vi "OpenCVCam_Close.vi"(8 "ErrorIn":errorcluster, 10 "CmdData":variant, 11 "OpenCVCamIn":refnum<class>) -> (0 "ErrorOut":errorcluster, 2 "ReplyData":variant, 3 "OpenCVCamOut":refnum<class>, 4 "Exit":bool)   [LabVIEW 2021, in "OpenCVCam.lvclass"]
uses:
  OpenCVCam.lvclass
  OpenCVCam.lvclass/OpenCVCam.ctl
  State.ctl
  C:/Localdata/Projects/TriekselSoft/TriekselsoftApplicationFramework/Source/.Externals/Library_EmguCV/Emgu.CV.Platform.NetStandard.dll
  Library_EmguCV/Emgu.CV.Platform.NetStandard.dll
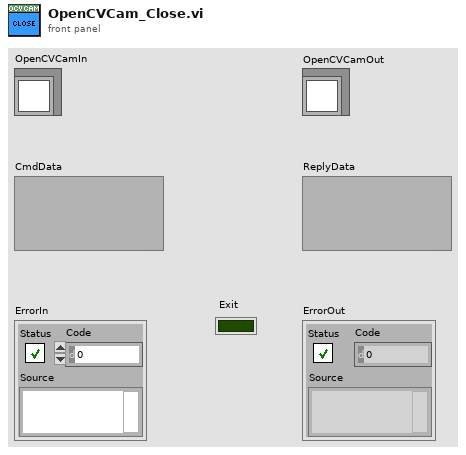
[diagram p1: front panel]
types:
  T1 = typedef "OpenCVCam.lvclass/State.ctl" = enum16{"Idle", "Initialized", "Acquiring"}
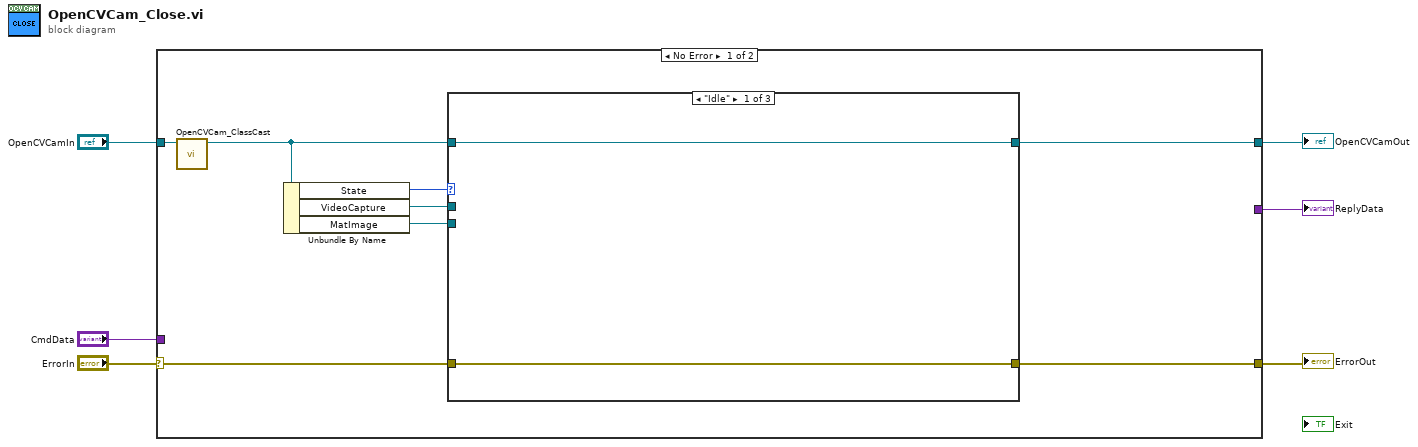
[diagram p0: block diagram]
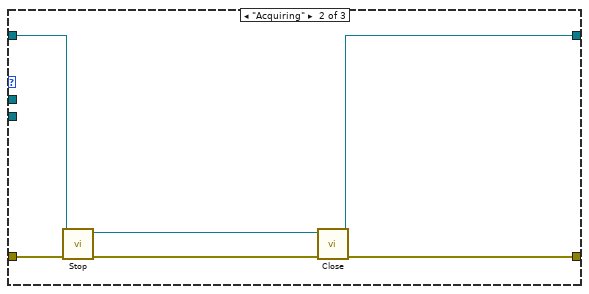
[diagram p2: hidden frame]
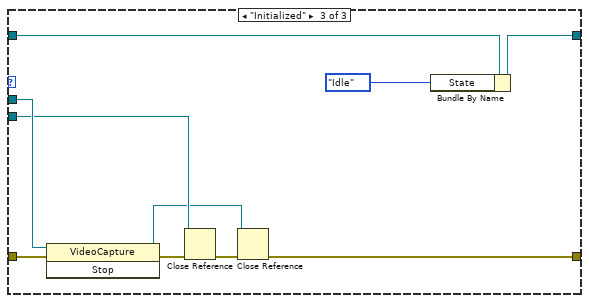
[diagram p3: hidden frame]
diagram:
  n1 = case shown="No Error" "ErrorIn" {
    selector: "ErrorIn" -> [w14 w35]
    tunnel: [w13 w35] -> w5
    tunnel: [_ w34] -> w3
    tunnel: "CmdData" -> [_ w34]
    tunnel: "OpenCVCamIn" -> [w12 w33]
    tunnel: [w7 w33] -> w1
    frame No Error {
      n2 = call "OpenCVCam_ClassCast.vi"("OpenCVCamIn"=w12) -> ("OpenCVCamOut"=w8:refnum<class "OpenCVCam.lvclass">)  [unwired: 10 in]
      n3 = Unbundle By Name(w8) -> ("State"=w11:T1, "VideoCapture"=w10:refnum<k24>, "MatImage"=w9:refnum<k24>)
      n4 = case shown="\"Idle\"" w11 {
        tunnel: [w16 w20 w31] -> w13
        tunnel: w14 -> [w16 w22 w29]
        tunnel: w10 -> [_ _ w28]
        tunnel: w9 -> [_ _ w27]
        tunnel: w8 -> [w15 w19 w25]
        tunnel: [w15 w17 w24] -> w7
        frame "Idle" {
        }
        frame "Acquiring" {
          n5 = call-dynamic "Stop.vi"("ErrorIn"=w22, "OpenCVCamIn"=w19) -> ("ErrorOut"=w21:errorcluster, "OpenCVCamOut"=w18:refnum<class "OpenCVCam.lvclass">)  [unwired: 8 in]
          n6 = call-dynamic "Close.vi"("ErrorIn"=w21, "OpenCVCamIn"=w18) -> ("ErrorOut"=w20:errorcluster, "OpenCVCamOut"=w17:refnum<class "OpenCVCam.lvclass">)  [unwired: 8 in]
        }
        frame "Initialized" {
          n7 = invoke class="VideoCapture" method="Stop"(reference=w28, error in=w29) -> (reference out=w26:refnum<k24>, error out=w30:errorcluster)  [unwired: 1 in, 1 out]
          n8 = Close Reference(reference=w27, error in (no error)=w30) -> (error out=w32:errorcluster)
          n9 = Close Reference(reference=w26, error in (no error)=w32) -> (error out=w31:errorcluster)
          n10 = Bundle By Name(cluster=w25, "State"=State."Idle") -> (w24:refnum<class "OpenCVCam.lvclass">)
        }
      }
    }
    frame Error {
    }
  }
  "ErrorOut" <- w5
  "OpenCVCamOut" <- w1
  "ReplyData" <- w3
